vi "Response Message.vi"(8 "error in (no error)":errorcluster, 9 "Response Message Data":variant, 10 "Response Message":string, 11 "Process In":refnum<class "Process.lvclass">) -> (0 "error out":errorcluster, 3 "Process Out":refnum<class "Process.lvclass">)   [LabVIEW 2020, in "Process.lvclass"]
doc: "Respond to a request message. The response will only be delivered to the requesting method and. \nThis VI may only be called from within the same case of the Handle Messages VI which handles the request or from a Helper Loop or Asynchronous Action launched from the specific case."
uses:
  Process.lvclass
  Process.lvclass/Process.ctl
  Request Message Cluster.ctl
  <vilib>/Utility/error.llb/Clear Errors.vi
  <vilib>/Utility/error.llb/Error Cluster From Error Code.vi
  <vilib>/ErrorRing/Error Ring.xnode
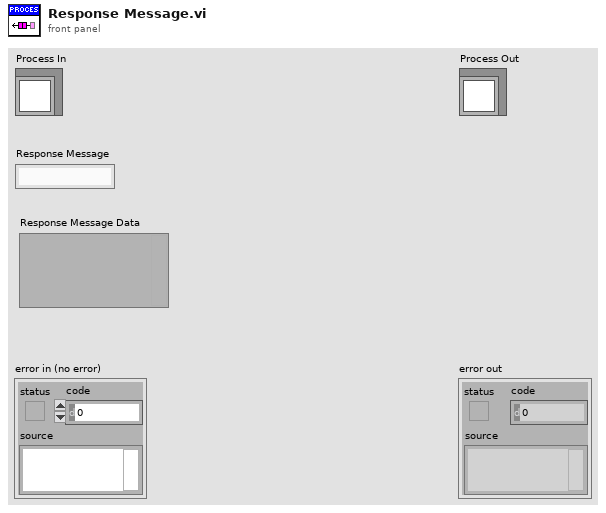
[diagram p1: front panel]
types:
  T1 = typedef "Process.lvclass/Request Message Cluster.ctl" = cluster{"Message":string, "Message Data":variant}
  T2 = typedef "Process.lvclass/Lifecycle State.ctl" = enum16{"Uninitialized", "Initialized", "Started", "Running", "Stopped", "Finished"}
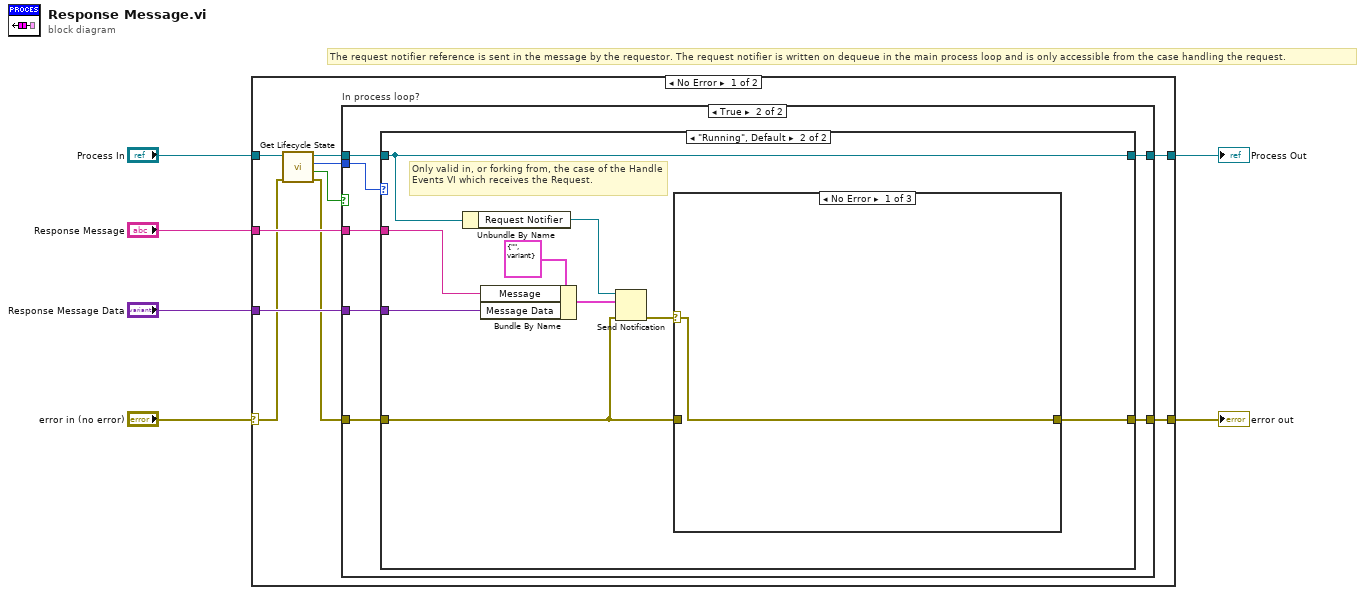
[diagram p0: block diagram]
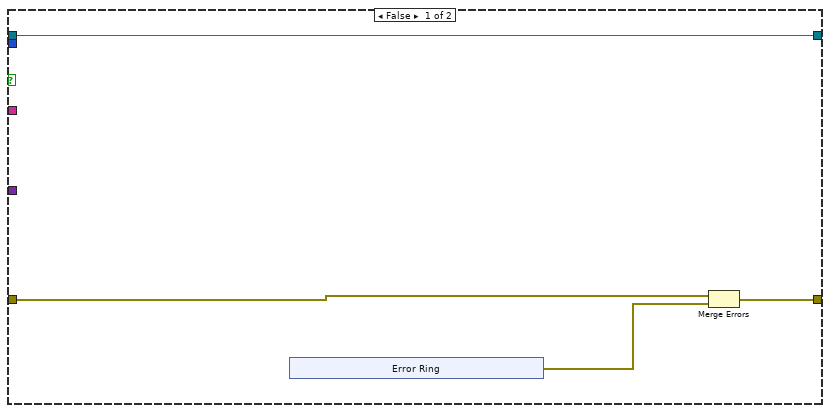
[diagram p2: hidden frame]
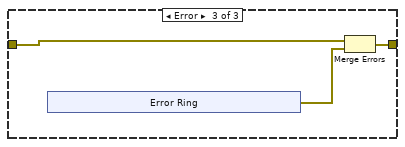
[diagram p5: hidden frame]
diagram:
  # "The request notifier reference is sent in the message by the requestor. The request notifier is written on dequeue in the main process loop and is only accessible from the case handling the request."
  n1 = case shown="No Error" "error in (no error)" {
    selector: "error in (no error)" -> [w11 w53]
    tunnel: "Process In" -> [w13 w52]
    tunnel: "Response Message" -> [w16 _]
    tunnel: "Response Message Data" -> [w15 _]
    tunnel: [w14 w53] -> w2
    tunnel: [w8 w52] -> w1
    frame No Error {
      n2 = call "Get Lifecycle State.vi"("error in (no error)"=w11, "Process In"=w13) -> ("error out"=w10:errorcluster, "In Process Loop?"=w7:bool, "Lifecycle State"=w9:T2, "Process Out"=w12:refnum<class "Process.lvclass">)  [unwired: 6 in]
      n3 = case "In process loop?" shown="True" w7 {
        tunnel: w16 -> [_ w31]
        tunnel: w15 -> [_ w30]
        tunnel: [w19 w29] -> w14
        tunnel: w12 -> [w20 w28]
        tunnel: w10 -> [w18 w27]
        tunnel: w9 -> [_ w26]
        tunnel: [w20 w25] -> w8
        frame False {
          n4 = xnode "Error Ring"() -> ("error out"=w17:errorcluster)
          n5 = Merge Errors(w18, w17) -> (w19:errorcluster)
        }
        frame True {
          n6 = case shown="\"Running\", Default" w26 {
            tunnel: w31 -> [_ w39]
            tunnel: w30 -> [_ w38]
            tunnel: [w32 w36] -> w29
            tunnel: w28 -> [w33 w35]
            tunnel: w27 -> [w32 w34]
            tunnel: [w33 w35] -> w25
            frame "Stopped" {
              # "If the process is stopped, the wait for reply VI will abort and throw an error. \nThere is no reason to throw an error here as well."
            }
            frame "Running", Default {
              # "Only valid in, or forking from, the case of the Handle Events VI which receives the Request."
              n7 = Unbundle By Name(w35) -> ("Request Notifier"=w42:refnum<notifier>)
              n8 = Bundle By Name(cluster=T1 {"Message"="", "Message Data"=variant} ("notification"), "Message"=w39, "Message Data"=w38) -> (w40:T1)
              n9 = Send Notification(notification=w40, notifier=w42, error in (no error)=w34) -> (error out=w37:errorcluster)  [unwired: 1 out]
              n10 = case shown="No Error" w37 {
                selector: w37 -> [w43 w44 _]
                tunnel: [w43 w44 w46] -> w36
                tunnel: w34 -> [_ _ w45]
                frame No Error {
                }
                frame Default {
                }
                frame Error {
                  n11 = xnode "Error Ring"() -> ("error out"=w47:errorcluster)
                  n12 = Merge Errors(w45, w47) -> (w46:errorcluster)
                }
              }
            }
          }
        }
      }
    }
    frame Error {
    }
  }
  "error out" <- w2
  "Process Out" <- w1
